vi "Read initialTime.vi"(8 "error in (no error)":errorcluster, 11 "ElectrometerController in":refnum<class "ElectrometerController.lvclass">) -> (0 "error out":errorcluster, 2 "initialTime":dbl, 3 "ElectrometerController out":refnum<class "ElectrometerController.lvclass">)   [LabVIEW 2016, in "ElectrometerController.lvclass"]
uses:
  ElectrometerController.lvclass
  ElectrometerController.lvclass/ElectrometerController.ctl
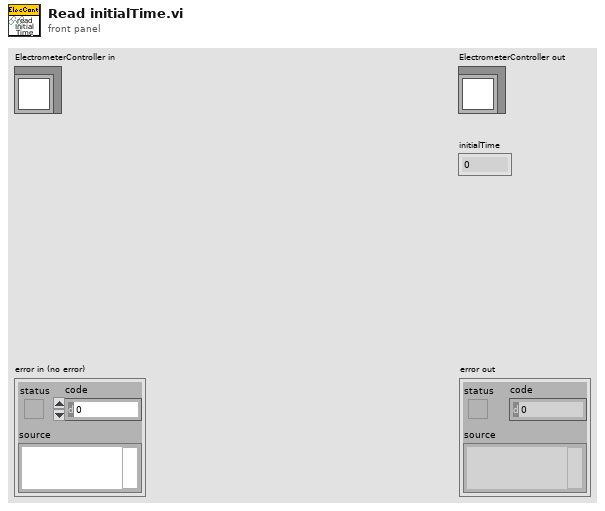
[diagram p1: front panel]
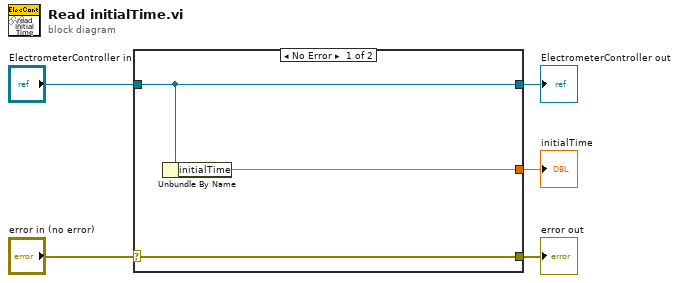
[diagram p0: block diagram]
diagram:
  n1 = case shown="No Error" "error in (no error)" {
    selector: "error in (no error)" -> [w8 w9]
    tunnel: [w8 w9] -> w4
    tunnel: [w7 w10] -> w2
    tunnel: "ElectrometerController in" -> [w7 w10]
    tunnel: [w6 _] -> w1
    frame No Error {
      n2 = Unbundle By Name(w7) -> ("initialTime"=w6:dbl)
    }
    frame Error {
    }
  }
  "error out" <- w4
  "ElectrometerController out" <- w2
  "initialTime" <- w1
